vi "Event Message Errors.vi"(8 "error in":errorcluster) -> (0 "error out":errorcluster)   [LabVIEW 2020, in "Manager.lvlib"]
uses:
  Manager.lvlib
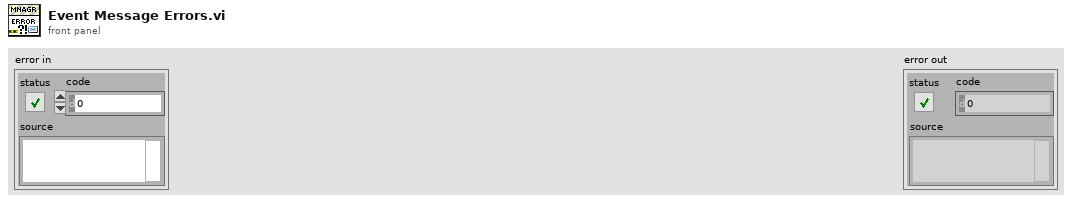
[diagram p1: front panel]
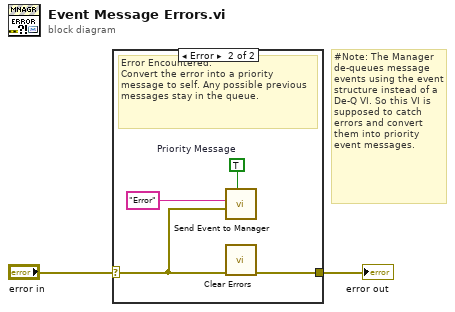
[diagram p0: block diagram]
diagram:
  # "#Note: The Manager de-queues message events using the event structure instead of a De-Q VI. So this VI is supposed to catch errors and convert them into priority event messages."
  n1 = case shown="Error" "error in" {
    selector: "error in" -> [w3 w4]
    tunnel: [w3 w7] -> w1
    frame No Error {
      # "No Error: Do nothing."
    }
    frame Error {
      w6 = TRUE  # Priority Message
      # "Error Encountered.\nConvert the error into a priority message to self. Any possible previous messages stay in the queue."
      n2 = call "Send Event to Manager.vi"("Priority Message"=w6, "Payload"=w4, "Command"="Error") -> ()  [unwired: 8 in, 1 out]
      n3 = call <vilib>:"Clear Errors.vi"("error in (no error)"=w4) -> ("error out"=w7:errorcluster)  [unwired: 5 in, 1 out]
    }
  }
  "error out" <- w1
